vi "20180223_test.vi"() -> ()   [LabVIEW 2014]
panel:
  out "Data Written":bool
  out "Data":u16 format="%.0x"
  out "error out":errorcluster
  in  "Address (0x50)":u16=80 max=1023 format="%.0x"
  in  "error in (no error)":errorcluster
  out "Bit Rate":i16
  out "Aardvark Power Enable":bool
  out "Pullup?":bool
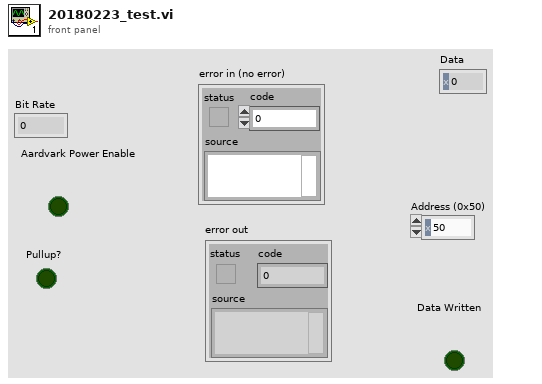
[diagram p1: front panel]
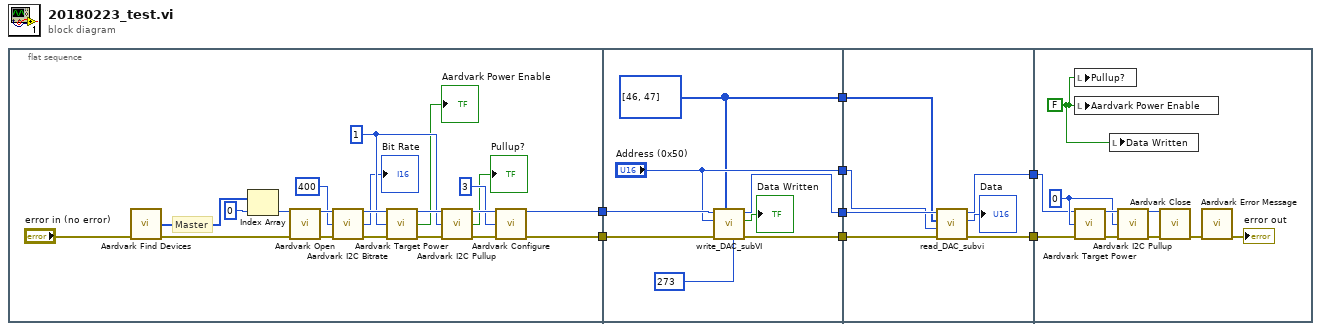
[diagram p0: block diagram]
diagram:
  n1 = flat-sequence {
    tunnel: [w10] -> w6
    tunnel: [w9] -> w4
    tunnel: w6 -> [w33]
    tunnel: [w34] -> w5
    tunnel: w4 -> [w37]
    tunnel: [w36] -> w3
    tunnel: ["Address (0x50)"] -> w2
    tunnel: [w31] -> w1
    tunnel: w5 -> [w44]
    tunnel: [w43] -> w8
    tunnel: w3 -> [w41]
    tunnel: [w40] -> w7
    tunnel: w2 -> [w39]
    tunnel: w1 -> [w38]
    tunnel: w8 -> [w48]
    tunnel: w7 -> [w47]
    frame #0 {
      w15 = 1
      # "Master"
      n2 = call <instrlib>:"Aardvark Find Devices.vi"("error in (no error)"="error in (no error)") -> ("Ports"=w28:u16[], "error out"=w27:errorcluster)  [unwired: 12 in, 1 out]
      n3 = Index Array(array=w28, index=0) -> (element=w26:u16)
      n4 = call <instrlib>:"Aardvark Open.vi"("Port Number (0)"=w26, "error in (no error)"=w27) -> ("Aardvark Handle"=w24:i32, "error out"=w20:errorcluster)  [unwired: 12 in]
      n5 = call <instrlib>:"Aardvark I2C Bitrate.vi"("Aardvark Handle"=w24, "Requested Bitrate kHz (100)"=400, "error in (no error)"=w20) -> ("dup Aardvark Handle"=w23:i32, "Actual Bitrate kHz"=→"Bit Rate":i32, "error out"=w19:errorcluster)  [unwired: 10 in]
      n6 = call <instrlib>:"Aardvark Target Power.vi"("Aardvark Handle"=w23, "Requested Configuration (2: Query)"=w15, "error in (no error)"=w19) -> ("dup Aardvark Handle"=w22:i32, "Target Power Enabled?"=→"Aardvark Power Enable":bool, "error out"=w18:errorcluster)  [unwired: 10 in]
      n7 = call <instrlib>:"Aardvark I2C Pullup.vi"("Aardvark Handle"=w22, "Requested Configuration (query)"=w15, "error in (no error)"=w18) -> ("dup Aardvark Handle"=w21:i32, "Pullups Enabled?"=→"Pullup?":bool, "error out"=w17:errorcluster)  [unwired: 10 in]
      n8 = call <instrlib>:"Aardvark Configure.vi"("Aardvark Handle"=w21, "Requested Configuration (0x80: Query)"=3, "error in (no error)"=w17) -> ("dup Aardvark Handle"=w10:i32, "error out"=w9:errorcluster)  [unwired: 10 in, 1 out]
    }
    frame #1 {
      w31 = u16[] [46, 47]
      n9 = call "write_DAC_subVI.vi"("Aardvark Handle in"=w33, "Address (0x50) in"="Address (0x50)", "error in (no error)"=w37, "DAC_ADD"=w31, "DAC_Val"=u16 273) -> ("Dup Aardvark Handle"=w34:i32, "DAC Written"=→"Data Written":bool, "error out"=w36:errorcluster)  [unwired: 3 in]
    }
    frame #2 {
      n10 = call "read_DAC_subvi.vi"("error in (no error)"=w41, "Address (0x50)"=w39, "DAC_ADD"=w38, "Aardvark Handle"=w44) -> ("error out"=w40:errorcluster, "DAC Val"=→"Data":u16, "Dup Aardvark Handle"=w43:i32)  [unwired: 3 in]
    }
    frame #3 {
      w45 = FALSE
      w49 = 0
      n11 = local write "Pullup?"(w45) -> ()
      n12 = local write "Aardvark Power Enable"(w45) -> ()
      n13 = call <instrlib>:"Aardvark Target Power.vi"("Aardvark Handle"=w48, "Requested Configuration (2: Query)"=w49, "error in (no error)"=w47) -> ("dup Aardvark Handle"=w52:i32, "error out"=w50:errorcluster)  [unwired: 10 in, 1 out]
      n14 = local write "Data Written"(w45) -> ()
      n15 = call <instrlib>:"Aardvark I2C Pullup.vi"("Aardvark Handle"=w52, "Requested Configuration (query)"=w49, "error in (no error)"=w50) -> ("dup Aardvark Handle"=w51:i32, "error out"=w46:errorcluster)  [unwired: 10 in, 1 out]
      n16 = call <instrlib>:"Aardvark Close.vi"("Aardvark Handle"=w51, "error in (no error)"=w46) -> ("error out"=w53:errorcluster)  [unwired: 13 in]
      n17 = call <instrlib>:"Aardvark Error Message.vi"("error in (no error)"=w53) -> ("error out"=→"error out":errorcluster)  [unwired: 10 in, 4 out]
    }
  }
